vi "GetObjectConfiguration.vi"(8 "Error In":errorcluster) -> (0 "Error Out":errorcluster)   [LabVIEW 2021, in "Application.lvclass"]
uses:
  Application.lvclass
  Interface_TAF_IApplicationConfiguration/IApplicationConfiguration/IApplicationConfiguration.lvclass
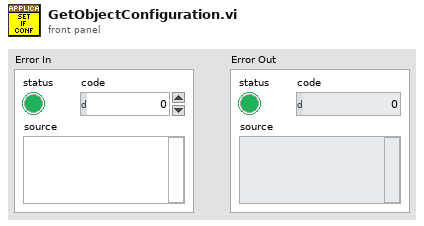
[diagram p1: front panel]
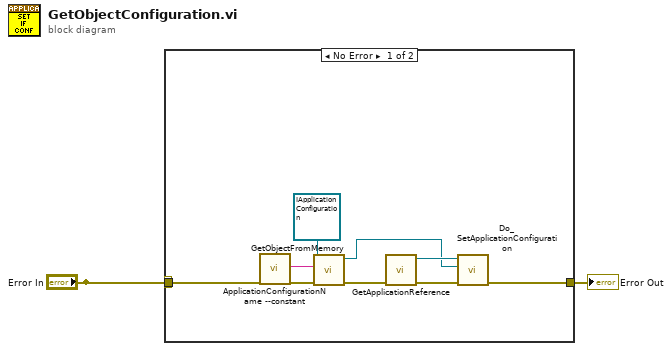
[diagram p0: block diagram]
diagram:
  n1 = case shown="No Error" "Error In" {
    selector: "Error In" -> [w5 w11]
    tunnel: [w8 w11] -> w2
    tunnel: "Error In" -> [_ _]
    frame No Error {
      n2 = call "ApplicationConfigurationName --constant.vi"() -> ("AppConfigName"=w6:string)  [unwired: 10 in, 1 out]
      n3 = call "GetObjectFromMemory.vi"("error in (no error)"=w5, "ObjectName"=w6, "Type"=refnum<class "IApplicationConfiguration.lvclass"> refnum ("IApplicationStructure")) -> ("error out"=w4:errorcluster, "ObjectOut"=w3:refnum<class "IApplicationConfiguration.lvclass">)  [unwired: 7 in]
      n4 = call "GetApplicationReference.vi"("error in (no error)"=w4) -> ("error out"=w10:errorcluster, "Application out"=w9:refnum<class "Application.lvclass">)  [unwired: 9 in]
      n5 = call-dynamic "Do_SetApplicationConfiguration.vi"("Error In"=w10, "ConfigSource"=w3, "ApplicationIn"=w9) -> ("Error Out"=w8:errorcluster)  [unwired: 6 in, 2 out]
    }
    frame Error {
    }
  }
  "Error Out" <- w2
